vi "Keyence_读取单个寄存器数据.vi"(0 "Keyence ID In":refnum<k5>, 1 "Delay Time (s)":dbl=1.0 caption="延迟时间(s)", 5 "软元件编号":string, 11 "错误输入（无错误）":errorcluster) -> (4 "Keyence ID Out":refnum<k5>, 6 "数据输出":string, 10 "状态":bool, 15 "错误输出":errorcluster)   [LabVIEW 2017]
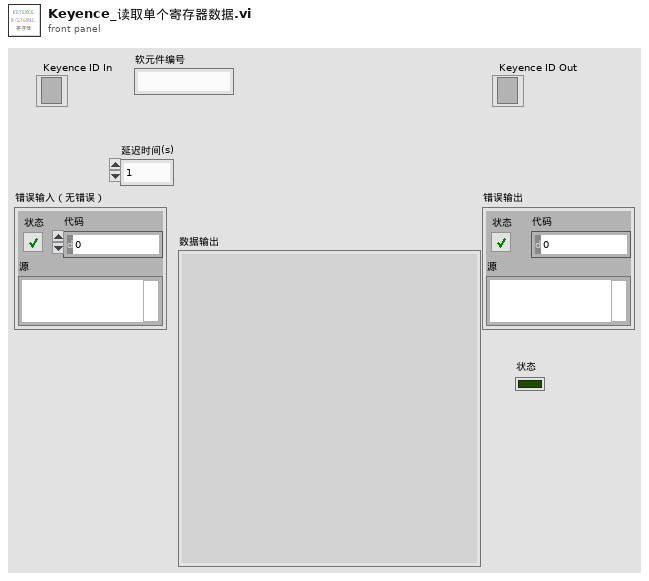
[diagram p1: front panel]
types:
  T1 = enum16{"Standard", "Buffered", "CRLF", "Immediate"}
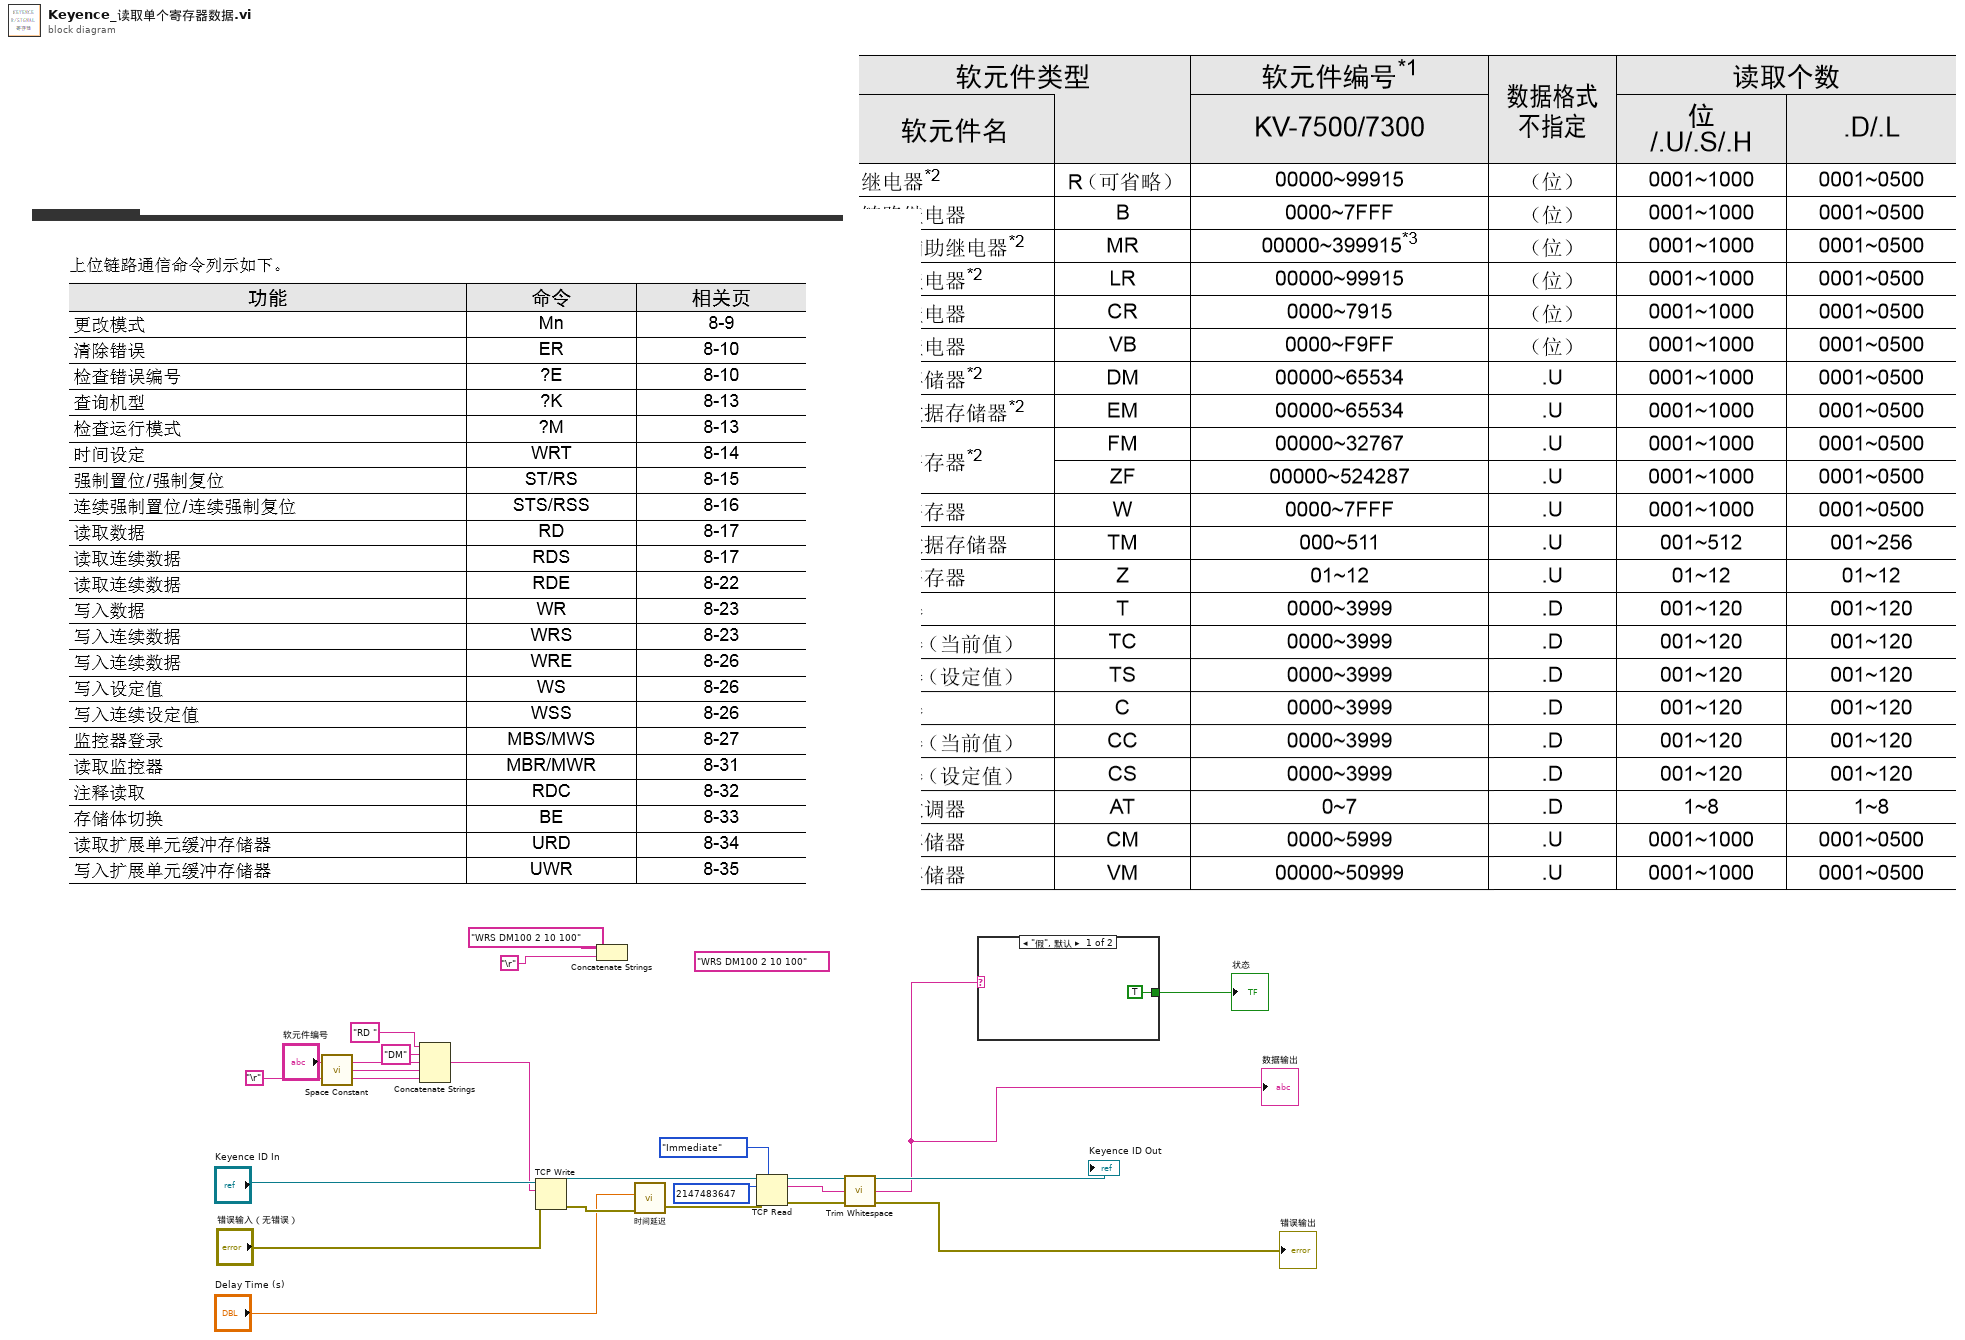
[diagram p0: block diagram]
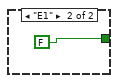
[diagram p2: hidden frame]
diagram:
  (unwired) "WRS DM100 2 10 100"
  n1 = call <vilib>:"Space Constant.vi"() -> ("String"=w8:string)
  n2 = Concatenate Strings("RD ", "DM" ("字符串"), "软元件编号", w8, "\r") -> (w6:string)
  n3 = TCP Write(connection ID="Keyence ID In", data in=w6, error in (no error)="错误输入（无错误）") -> (connection ID out=w19:refnum<k5>, error out=w18:errorcluster)  [unwired: 1 in, 1 out]
  n4 = Concatenate Strings("WRS DM100 2 10 100", "\r") -> ()  [unwired: 1 out]
  n5 = call "时间延迟"("error in (no error)"=w18, "Delay Time (s)"="Delay Time (s)") -> ("error out"=w13:errorcluster)  [unwired: 9 in]
  n6 = TCP Read(connection ID=w19, bytes to read=2147483647 ("读取的字节"), error in (no error)=w13, 7:T1."Immediate" ("模式（标准）")) -> (connection ID out=→"Keyence ID Out":refnum<k5>, data out=w3:string, error out=→"错误输出":errorcluster)  [unwired: 1 in]
  n7 = call <vilib>:"Trim Whitespace.vi"("string"=w3) -> ("trimmed string"=w2:string)  [unwired: 1 in]
  "数据输出" <- w2
  n8 = case shown="\"假\", 默认" w2 {
    tunnel: [TRUE FALSE] -> w1
    frame "假", Default {
    }
    frame "E1" {
    }
  }
  "状态" <- w1
